vi "2.1.vi"(1 "b":dbl, 2 "k":dbl, 3 "x":dbl) -> (0 "y":dbl)   [LabVIEW 2017]
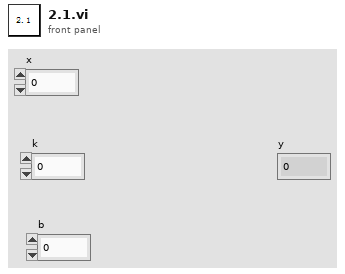
[diagram p1: front panel]
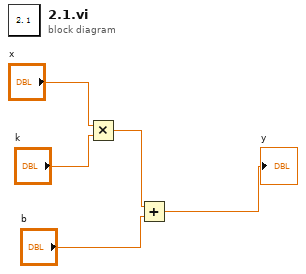
[diagram p0: block diagram]
diagram:
  n1 = Multiply(x="x", y="k") -> (x*y=w2:dbl)
  n2 = Add(x=w2, y="b") -> (x+y=→"y":dbl)
